vi "ErrorSubPanelVIMissing.vi"(0 "Create Error?":bool, 5 "VI Name":string, 11 "error in":errorcluster) -> (15 "error out":errorcluster)   [LabVIEW 2016]
doc: "Creates error if the VI is not found in the SubPanel"
uses:
  <vilib>/Utility/error.llb/Error Cluster From Error Code.vi
  <vilib>/ErrorRing/Error Ring.xnode
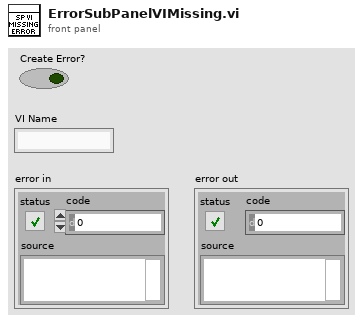
[diagram p1: front panel]
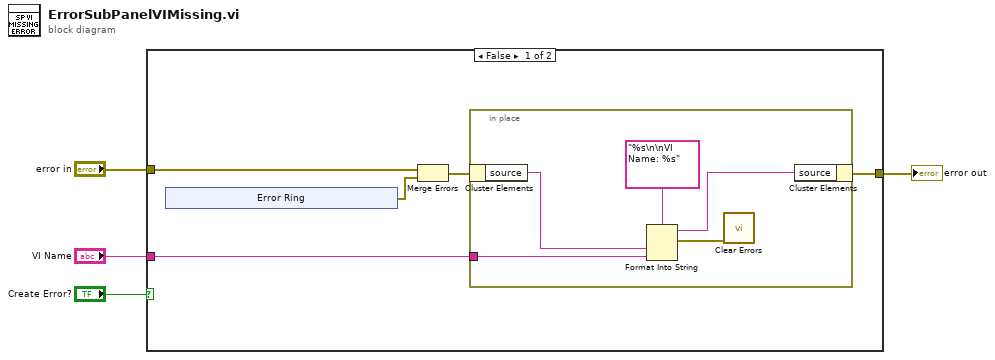
[diagram p0: block diagram]
diagram:
  n1 = case shown="False" "Create Error?" {
    tunnel: "error in" -> [w9 w20]
    tunnel: [w7 w20] -> w3
    tunnel: "VI Name" -> [w6 _]
    frame False {
      n2 = xnode "Error Ring"() -> ("error out"=w5:errorcluster)
      n3 = Merge Errors(w9, w5) -> (w8:errorcluster)
      n4 = in-place {
        in-place-border: w6 -> [w19]
        n5 = in-place-cluster #1(w8) -> ("source"=w16:string)
        n6 = Format Into String(format string="%s\n\nVI Name: %s", w16, w19) -> (resulting string=w17:string, error out=w15:errorcluster)  [unwired: 2 in]
        n7 = call <vilib>:"Clear Errors.vi"("error in (no error)"=w15) -> ()  [unwired: 5 in, 2 out]
        n8 = in-place-cluster #1("source"=w17) -> (w7:errorcluster)
      }
    }
    frame True {
    }
  }
  "error out" <- w3
